vi "Set Debug Mode.vi"(6 "clear debug data (F)":bool, 8 "error in":errorcluster, 10 "debug mode (F)":bool, 11 "GOLPI ref. in":T2={"pipe handle"={"lv_proc.dll file path"=path "", "process instance handle"=[], "debug mode"=FALSE, "debug data"=[]}, "fast read timeout [ms]"=500, "fast read settle time [ms]"=10, "fast read to multiple [ms]"=1, "max elements per input line"=100, "slow read timeout [ms]"=5000, "stdin double format specifier"="", "max elements per stdout output column"=100, "console mode bitstream"=FALSE, "bitstream first read timeout [ms]"=1000, "bitstream read timeout [ms]"=50, "struct transfer possible"=FALSE, "matlab mode"=FALSE}) -> (0 "error out":errorcluster, 1 "debug data strings concatenated":string, 2 "debug data":T1(array[cluster]), 3 "GOLPI ref. out":T2={"pipe handle"={"lv_proc.dll file path"=path "", "process instance handle"=[], "debug mode"=FALSE, "debug data"=[]}, "fast read timeout [ms]"=500, "fast read settle time [ms]"=10, "fast read to multiple [ms]"=1, "max elements per input line"=100, "slow read timeout [ms]"=5000, "stdin double format specifier"="", "max elements per stdout output column"=100, "console mode bitstream"=FALSE, "bitstream first read timeout [ms]"=1000, "bitstream read timeout [ms]"=50, "struct transfer possible"=FALSE, "matlab mode"=FALSE})   [LabVIEW 2020, in "GOLPI library.lvlib"]
doc: "Sets Debug mode of the LV Process library. If set, all stdin and stdout buffers are stored in GOLPI reference. Debug data can be retrieved again by this vi. (Internaly this vi only sets or reads data stored in GOLPI reference).\nDebug mode is usefull for watching all commands written into GNU Octave and reading all outputs, however it can take a lot of memory if used for a long time.\n\n---\nGOLPI works only with lv_proc.dll library, which is part of vipm package or should be delivered together with packed library. Placement of this dll is selected in terminal of Start GNU Octave.vi."
uses:
  GOLPI library.lvlib
  GOLPI reference Type Def.ctl
  Pipe Handle.ctl
  LV Process library.lvlib
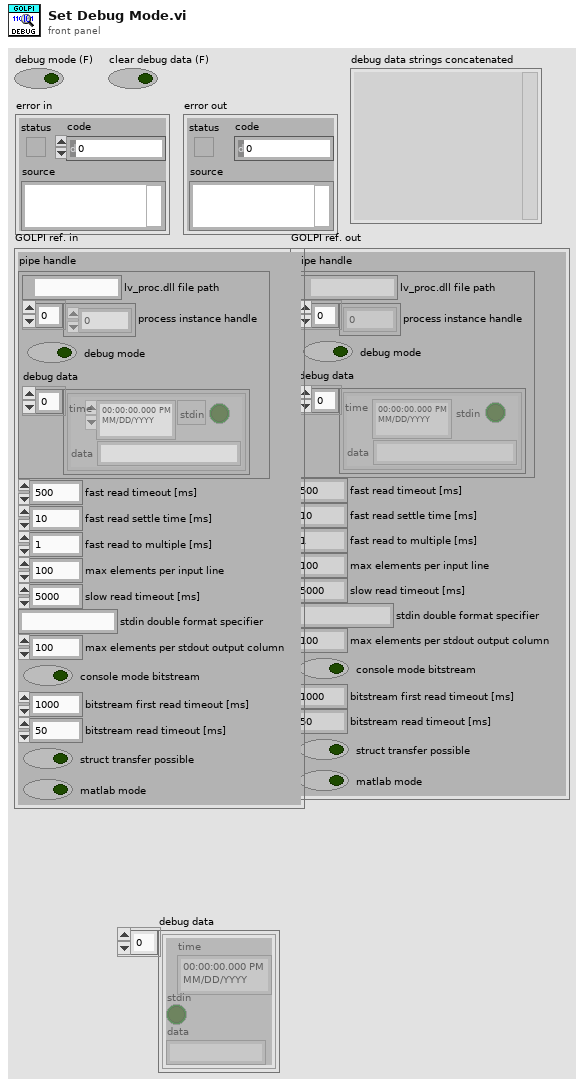
[diagram p1: front panel]
types:
  T1 = cluster{"time":timestamp, "stdin":bool, "data":string}[]
  T2 = typedef "GOLPI library.lvlib/GOLPI reference Type Def.ctl" = cluster{"pipe handle":T3, "fast read timeout [ms]":u32, "fast read settle time [ms]":u32, "fast read to multiple [ms]":u32, "max elements per input line":u32, "slow read timeout [ms]":u32, "stdin double format specifier":string, "max elements per stdout output column":u32, "console mode bitstream":bool, "bitstream first read timeout [ms]":u32, "bitstream read timeout [ms]":u32, "struct transfer possible":bool, "matlab mode":bool}
  T3 = typedef "LV Process library.lvlib/Pipe Handle.ctl" = cluster{"lv_proc.dll file path":path, "process instance handle":u32[], "debug mode":bool, "debug data":cluster{"time":timestamp, "stdin":bool, "data":string}[]}
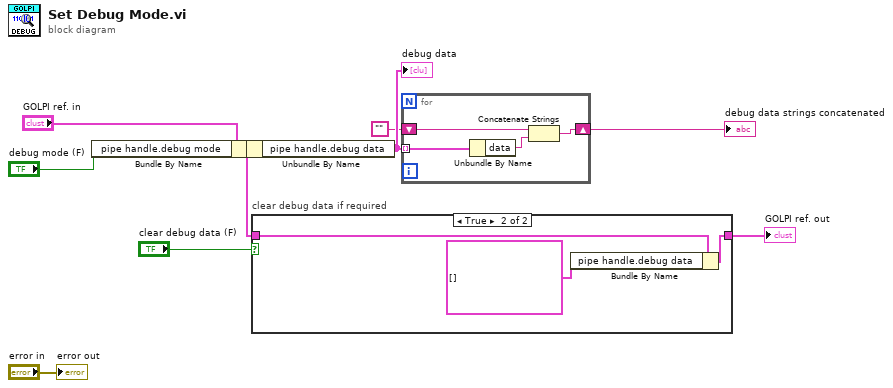
[diagram p0: block diagram]
diagram:
  n1 = Bundle By Name(cluster="GOLPI ref. in", "pipe handle.debug mode"="debug mode (F)") -> (w6:T2)
  n2 = Unbundle By Name(w6) -> ("pipe handle.debug data"=w3:T1)
  "debug data" <- w3
  n3 = case "clear debug data if required" shown="True" "clear debug data (F)" {
    tunnel: w6 -> [w10 w13]
    tunnel: [w10 w12] -> w4
    frame False {
    }
    frame True {
      n4 = Bundle By Name(cluster=w13, "pipe handle.debug data"=T1 []) -> (w12:T2)
    }
  }
  "GOLPI ref. out" <- w4
  n5 = for {
    tunnel: w3 -> [w17] mode=indexing
    shift-right: [w14] -> w1
    shift-left: "" -> [w15]
    n6 = Unbundle By Name(w17) -> ("data"=w16:string)
    n7 = Concatenate Strings(w15, w16) -> (w14:string)
  }
  "debug data strings concatenated" <- w1
  "error out" <- "error in"
